vi "ExampleInstrument.HELP.vi"(8 "error in (no error)":errorcluster, 11 "ExampleInstrument in":refnum<class "ExampleInstrument.lvclass">) -> (0 "error out":errorcluster, 2 "Commands":string[](array[string]), 3 "ExampleInstrument out":refnum<class "ExampleInstrument.lvclass">)   [LabVIEW 2016, in "ExampleInstrument.lvclass"]
uses:
  ExampleInstrument.lvclass
  C:/user/patrick/hg/levylab_inst/lvsrc/SMOs/Instrument/Instrument.lvclass
  SMOs/Instrument/Instrument.lvclass
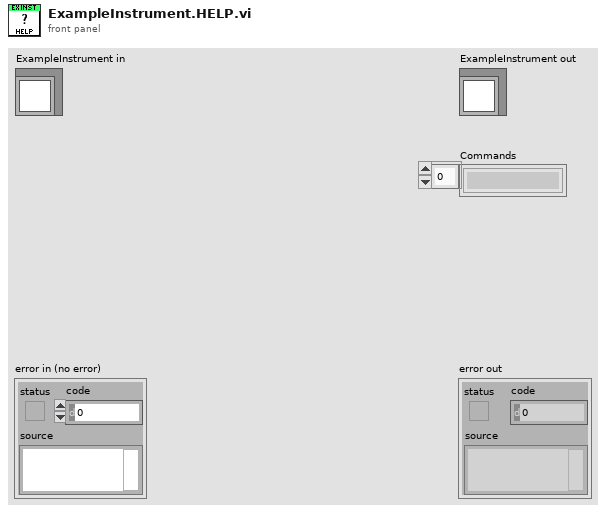
[diagram p1: front panel]
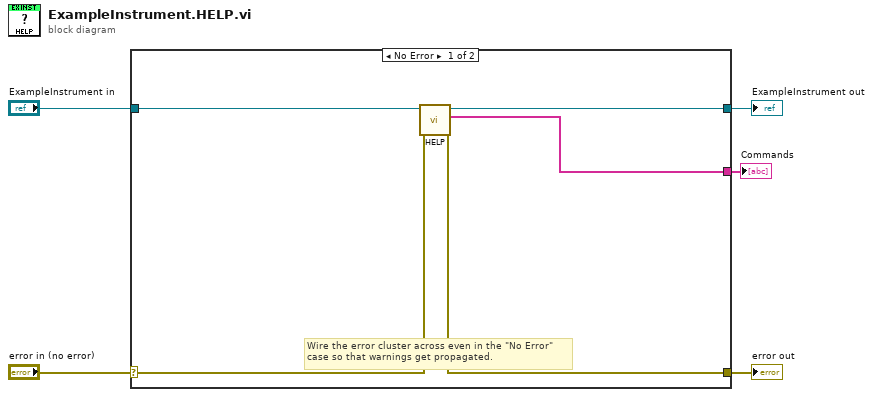
[diagram p0: block diagram]
diagram:
  n1 = case shown="No Error" "error in (no error)" {
    selector: "error in (no error)" -> [w8 w12]
    tunnel: [w6 w12] -> w4
    tunnel: [w9 w11] -> w2
    tunnel: "ExampleInstrument in" -> [w10 w11]
    tunnel: [w7 _] -> w1
    frame No Error {
      # "Wire the error cluster across even in the \"No Error\"\ncase so that warnings get propagated."
      n2 = call "HELP.vi"("error in (no error)"=w8, "Instrument in"=w10) -> ("error out"=w6:errorcluster, "Commands"=w7:string[], "Instrument out"=w9:refnum<class "ExampleInstrument.lvclass">)  [unwired: 7 in]
    }
    frame Error {
    }
  }
  "error out" <- w4
  "ExampleInstrument out" <- w2
  "Commands" <- w1
